vi "tdms2csv.vi"() -> ()   [LabVIEW 2017]
uses:
  <vilib>/Waveform/WDTFileIO.llb/Export Waveforms To Spreadsheet File (1D).vi
panel:
  out "waveform":dynamicdata(graph)
  in  "Stop":bool
  in  "start":bool
  in  "File path":path
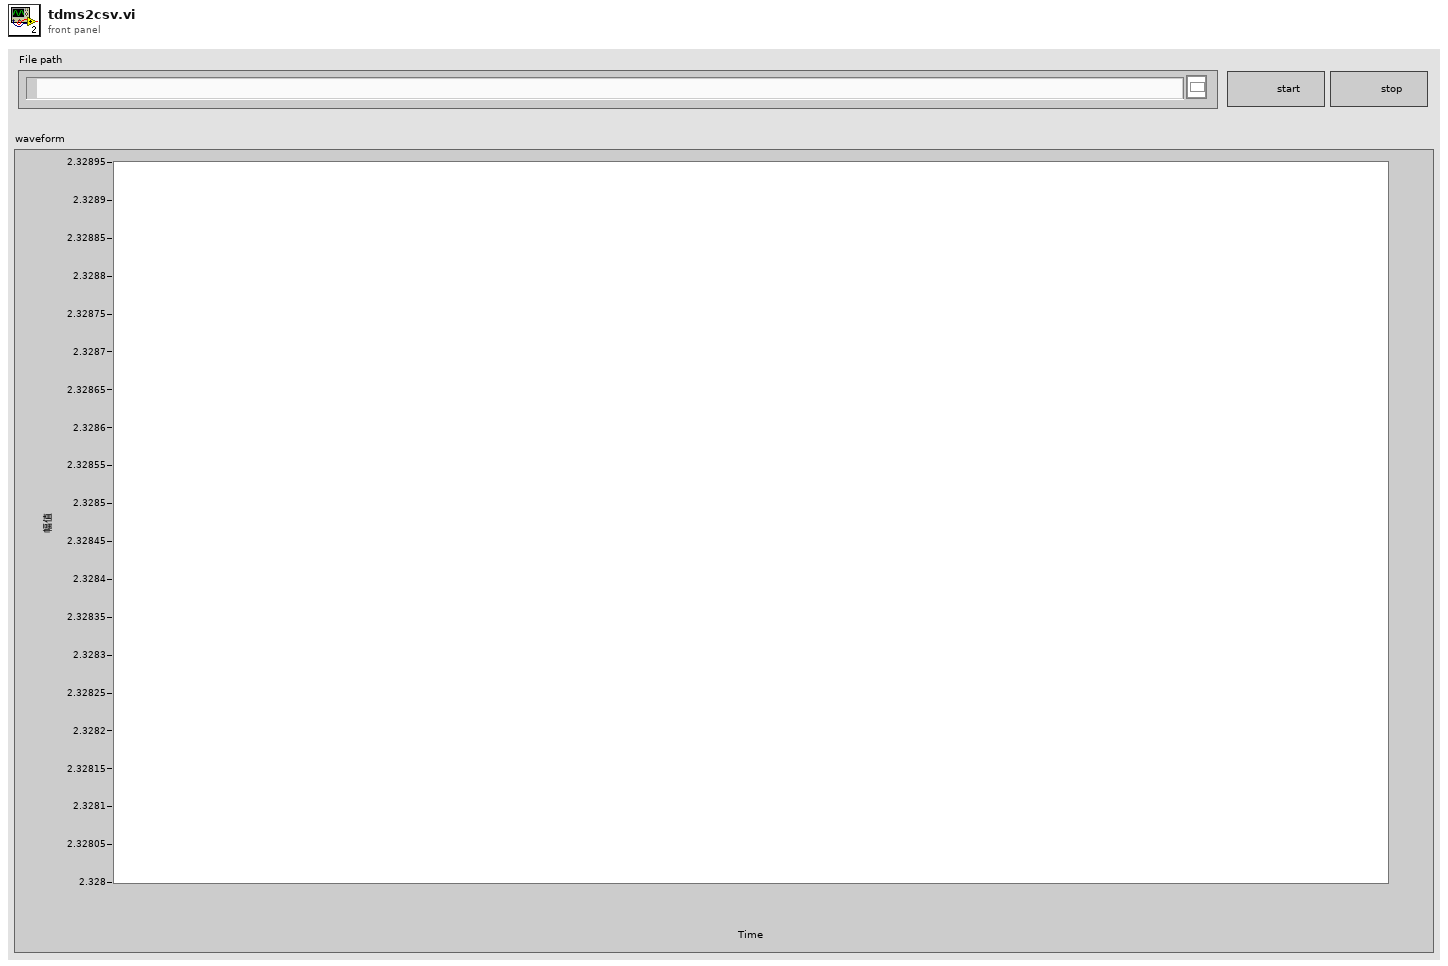
[diagram p1: front panel]
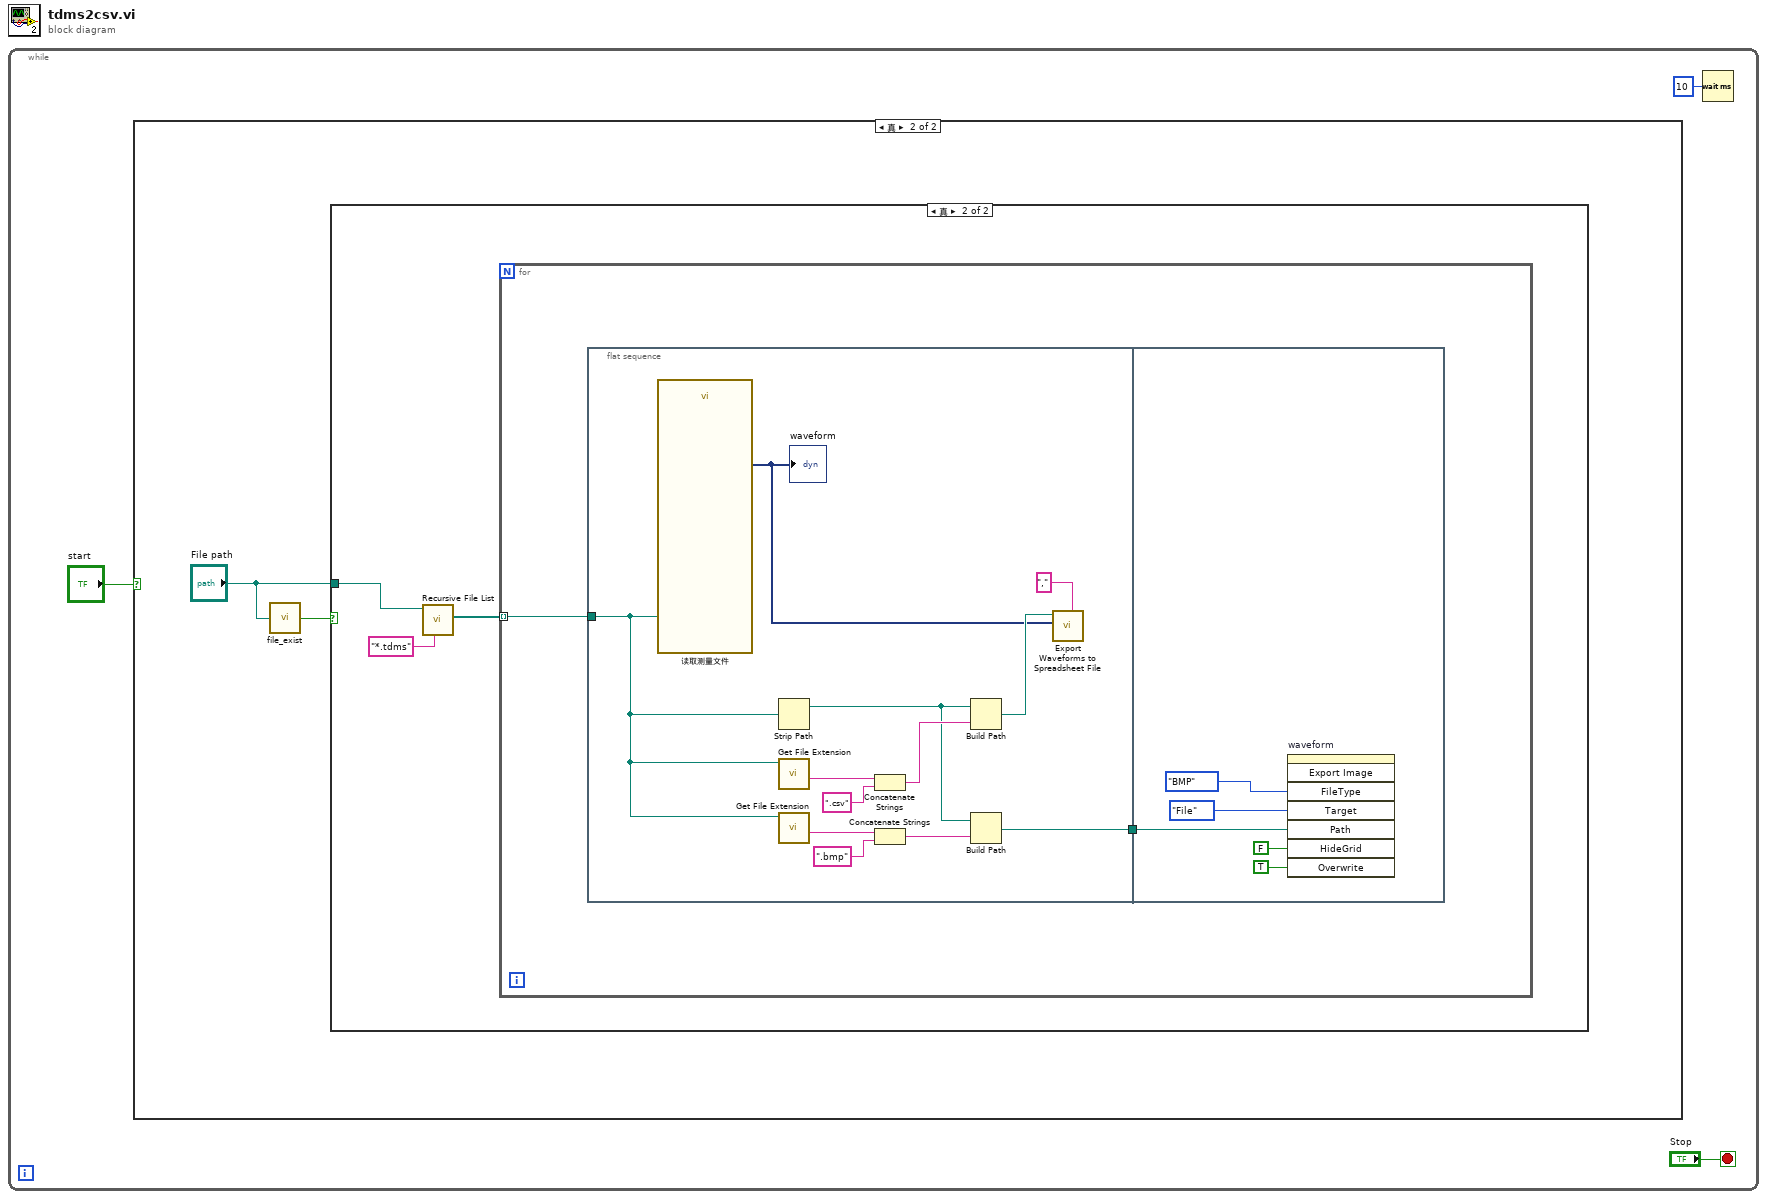
[diagram p0: block diagram]
diagram:
  n1 = while {
    stop <- "Stop" stop-if-true
    n2 = case shown="真" "start" {
      frame False {
      }
      frame True {
        n3 = call "file_exist.vi"("File path name input"="File path") -> ("File exist?"=w5:bool)
        n4 = case shown="真" w5 {
          tunnel: "File path" -> [_ w6]
          frame False {
          }
          frame True {
            n5 = call <vilib>:"Recursive File List.vi"("pattern"="*.tdms", "Folder Path"=w6) -> ("All Files in Dir"=w7:path[])  [unwired: 5 in, 4 out]
            n6 = for {
              tunnel: w7 -> [w10] mode=indexing
              n7 = flat-sequence {
                tunnel: w10 -> [w14]
                tunnel: [w11] -> w9
                tunnel: w9 -> [w25]
                frame #0 {
                  n8 = call "读取测量文件"("Filename"=w14) -> ("Signals"=w17:dynamicdata)  [unwired: 5 in, 5 out]
                  "waveform" <- w17
                  n9 = Strip Path(path=w14) -> (stripped path=w13:path)  [unwired: 1 out]
                  n10 = call <vilib>:"Get File Extension.vi"("file"=w14) -> ("filename without extension"=w21:string)  [unwired: 6 in, 4 out]
                  n11 = call <vilib>:"Get File Extension.vi"("file"=w14) -> ("filename without extension"=w15:string)  [unwired: 6 in, 4 out]
                  n12 = Concatenate Strings(w21, ".csv" ("字符串")) -> (w19:string)
                  n13 = Concatenate Strings(w15, ".bmp" ("字符串")) -> (w12:string)
                  n14 = Build Path(base path=w13, name or relative path=w19) -> (appended path=w18:path)
                  n15 = Build Path(base path=w13, name or relative path=w12) -> (appended path=w11:path)
                  n16 = call-poly <vilib>:"Export Waveforms to Spreadsheet File.vi"("delimiter (Tab)"=",", "waveforms"=w17, "file path (dialog if empty)"=w18) -> ()  [unwired: 7 in, 2 out]
                }
                frame #1 {
                  n17 = invoke on="waveform" class="WFChart (严格)" method="Export Image"("FileType"=enum32{"BMP", "EPS", "EMF", "PICT"}."BMP" ("文件类型"), "Target"=enum32{"File", "Clipboard"}."File" ("目标"), "Path"=w25, "HideGrid"=FALSE ("隐藏网格"), "Overwrite"=TRUE ("始终覆盖")) -> ()  [unwired: 3 in, 8 out]
                }
              }
            }
          }
        }
      }
    }
    n18 = Wait (ms)(milliseconds to wait=u32 10 ("等待时间（毫秒）")) -> ()  [unwired: 1 out]
  }
